vi "Trigger Prepare Event for Listen.vi"(8 "error in (no error)":errorcluster, 11 "CIFCorePlugin in":refnum<class "CIFCorePlugin.lvclass">) -> (0 "error out":errorcluster)   [LabVIEW 2021, in "CIFCorePlugin.lvclass"]
uses:
  CIFCorePlugin.lvclass
  CIFCorePlugin.lvclass/CIFCorePlugin.ctl
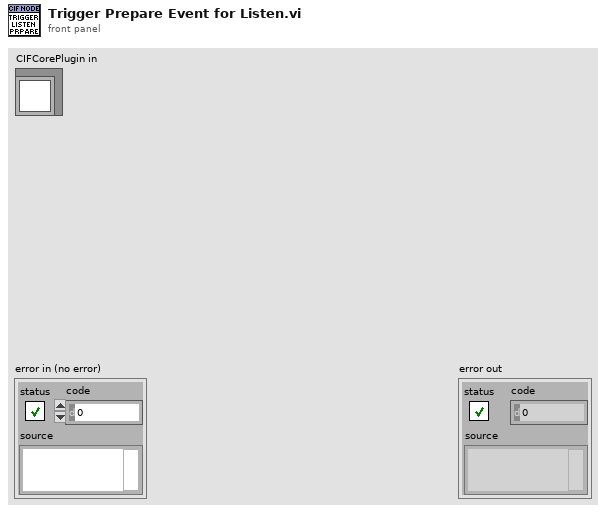
[diagram p1: front panel]
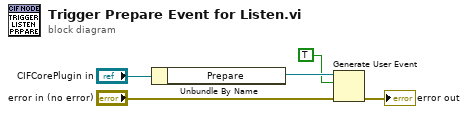
[diagram p0: block diagram]
diagram:
  n1 = Unbundle By Name("CIFCorePlugin in") -> ("Prepare"=w2:refnum<user-event>)
  n2 = Generate User Event(user event=w2, event data cluster=TRUE ("event data"), error in="error in (no error)") -> (error out=→"error out":errorcluster)  [unwired: 1 in, 1 out]
